vi "RenameClassSpecific.vi"(0 "ClassWriterGOOP300.lvclass":refnum<class "ClassWriterGOOP300.lvclass">, 1 "ClassRef":refnum<vi>, 2 "NewClassPath":path, 5 "error in":errorcluster) -> (14 "ClassWriterGOOP300.lvclass 2":refnum<class "ClassWriterGOOP300.lvclass">, 19 "error out":errorcluster)   [LabVIEW 2014, in "ClassWriterGOOP300.lvclass"]
uses:
  <resource>/Framework/Providers/Open_GDS/ClassProviders/Provider_EndevoGOOP300/ClassWriterGOOP300_class/ClassWriterGOOP300.lvclass
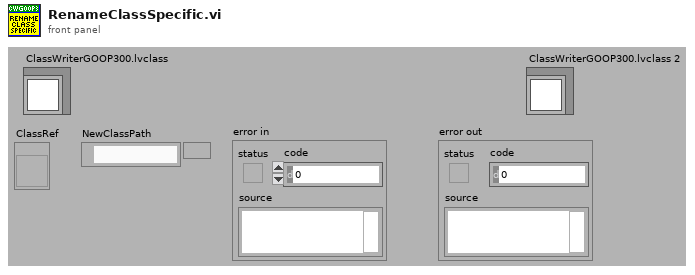
[diagram p1: front panel]
types:
  T1 = typedef "imagedata.ctl" = cluster{"image type":i32, "image depth":i32, "image":u8[], "mask":u8[], "colors":u32[], "Rectangle":cluster{"left":i16, "top":i16, "right":i16, "bottom":i16}}
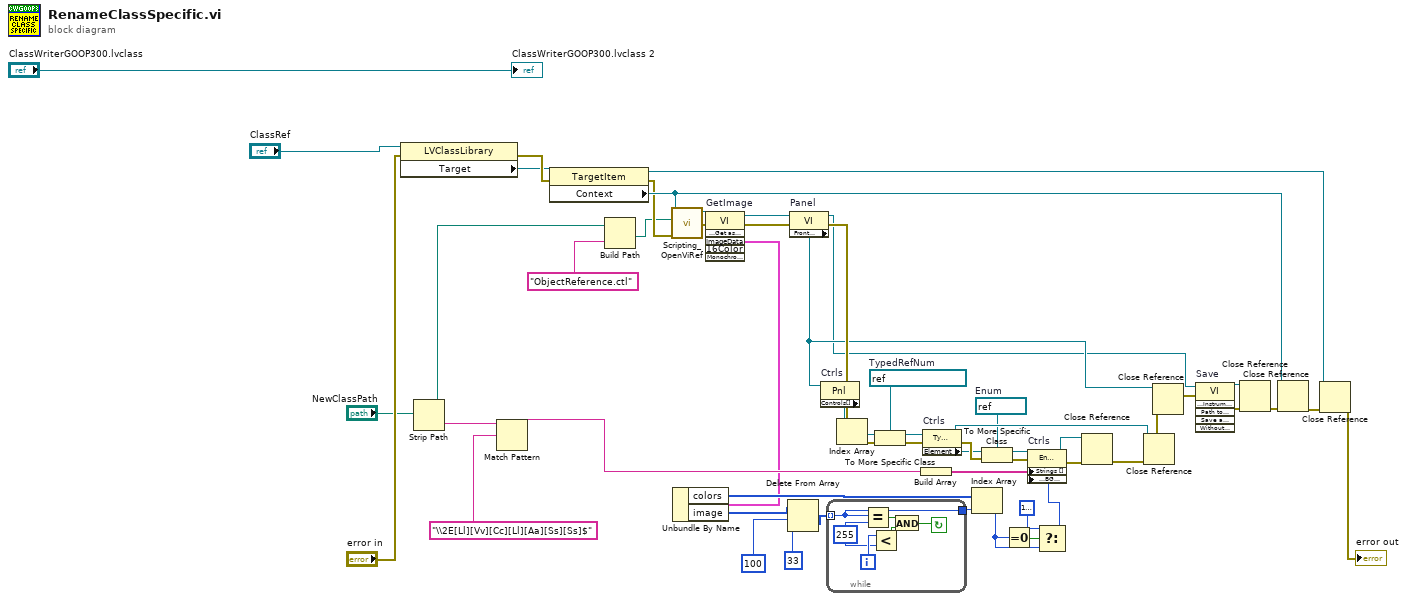
[diagram p0: block diagram]
diagram:
  w8 = refnum<vi> refnum  # Enum
  w5 = refnum<vi> refnum  # TypedRefNum
  n1 = property class="LVClassLibrary"(reference="ClassRef", error in="error in") -> (error out=w49:errorcluster, "Target"=w47:refnum<vi>)  [unwired: 1 out]
  n2 = Strip Path(path="NewClassPath") -> (stripped path=w45:path, name=w51:string)
  n3 = Match Pattern(string=w51, regular expression="\\2E[Ll][Vv][Cc][Ll][Aa][Ss][Ss]$" ("string")) -> (before substring=w52:string)  [unwired: 1 in, 3 out]
  n4 = property class="TargetItem"(reference=w47, error in=w49) -> (reference out=w55:refnum<vi>, error out=w37:errorcluster, "Context"=w43:refnum<vi>)
  n5 = Build Path(base path=w45, name or relative path="ObjectReference.ctl") -> (appended path=w36:path)
  n6 = call <resource>:"Scripting_OpenViRef.vi"("error in"=w37, "ViPath/ViName/Viref"=w36, "AppRef"=w43) -> ("error out"=w24:errorcluster, "vi reference"=w23:refnum<vi>)  [unwired: 6 in, 1 out]
  n7 = invoke on="GetImage" class="VI" method="VI Icon.Get as Image Data"(reference=w23, error in=w24) -> (reference out=w25:refnum<vi>, error out=w26:errorcluster, "ImageData"=w27:T1)  [unwired: 4 in, 3 out]
  n8 = Unbundle By Name(w27) -> ("colors"=w30:u32[], "image"=w28:u8[])
  n9 = Delete From Array(array=w28, length=100, index=33) -> (deleted portion=w38:u8[])  [unwired: 1 out]
  n10 = property on="Panel" class="VI"(reference=w25, error in=w26) -> (reference out=w19:refnum<vi>, error out=w41:errorcluster, "Front Panel"=w40:refnum<vi>)
  n11 = property on="Ctrls" class="Pnl"(reference=w40, error in=w41) -> ("Controls[]"=w3:refnum<vi>[])  [unwired: 2 out]
  n12 = while {
    tunnel: w38 -> [w56] mode=indexing
    tunnel: [w56] -> w39
    i -> [w60]
    stop <- w57 continue-if-true
    w59 = 255
    n13 = Equal?(x=w56, y=w59) -> (x = y?=w61:bool)
    n14 = Less?(x=w60, y=w59) -> (x < y?=w58:bool)
    n15 = And(x=w61, y=w58) -> (x .and. y?=w57:bool)
  }
  n16 = Index Array(array=w3) -> (element=w4:refnum<vi>)  [unwired: 1 in]
  n17 = To More Specific Class(target class=w5, reference=w4, error in=w41) -> (specific class reference=w6:refnum<vi>, error out=w11:errorcluster)
  n18 = Build Array(w52) -> (w10:string[])
  n19 = property on="Ctrls" class="TypRef"(reference=w6, error in=w11) -> (reference out=w17:refnum<vi>, error out=w12:errorcluster, "Element"=w7:refnum<vi>)
  n20 = Index Array(array=w30, index=w39) -> (element=w33:u32)
  n21 = To More Specific Class(target class=w8, reference=w7, error in=w12) -> (specific class reference=w9:refnum<vi>, error out=w13:errorcluster)
  n22 = Equal To 0?(x=w33) -> (x = 0?=w32:bool)
  n23 = Select(t=u32 16777216, s=w32, f=w33) -> (s? t:f=w34:u32)
  n24 = property on="Ctrls" class="Enum"(reference=w9, error in=w13, "Strings []"=w10, "Named Numeric Colors:BG Color"=w34) -> (reference out=w14:refnum<vi>, error out=w15:errorcluster)
  n25 = Close Reference(reference=w14, error in (no error)=w15) -> (error out=w16:errorcluster)
  n26 = Close Reference(reference=w17, error in (no error)=w16) -> (error out=w18:errorcluster)
  n27 = Close Reference(reference=w40, error in (no error)=w18) -> (error out=w20:errorcluster)
  n28 = invoke on="Save" class="VI" method="Save.Instrument"(reference=w19, error in=w20) -> (reference out=w21:refnum<vi>, error out=w22:errorcluster)  [unwired: 4 in, 4 out]
  n29 = Close Reference(reference=w21, error in (no error)=w22) -> (error out=w42:errorcluster)
  n30 = Close Reference(reference=w43, error in (no error)=w42) -> (error out=w53:errorcluster)
  n31 = Close Reference(reference=w55, error in (no error)=w53) -> (error out=→"error out":errorcluster)
  "ClassWriterGOOP300.lvclass 2" <- "ClassWriterGOOP300.lvclass"
